vi "Read U8.vi"(11 "unsigned byte array":u8[](array[numeric])) -> (3 "U8 Out":u8, 5 "rest of array":u8[](array[numeric]))   [LabVIEW 2015]
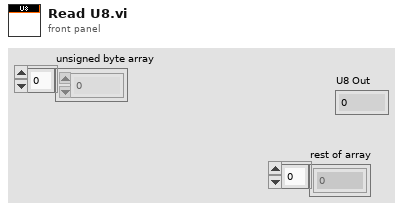
[diagram p1: front panel]
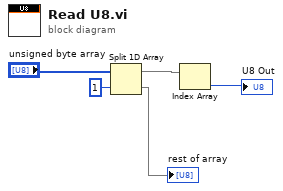
[diagram p0: block diagram]
diagram:
  n1 = Split 1D Array(array="unsigned byte array", index=1) -> (first subarray=w5:u8[], second subarray=→"rest of array":u8[])
  n2 = Index Array(array=w5) -> (element=→"U8 Out":u8)  [unwired: 1 in]
